vi "Create New Rubix Cube.vi"(8 "error out":errorcluster, 11 "Rubix Array pattern":string[][](array[string])) -> (0 "error out(no error)":errorcluster)   [LabVIEW 2019]
uses:
  Scene Commands.ctl
  Cube Data Ops.ctl
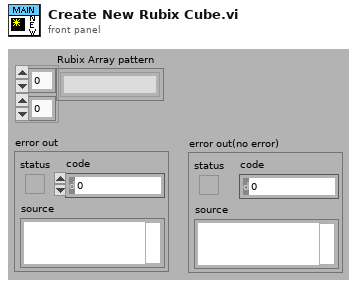
[diagram p1: front panel]
types:
  T1 = typedef "Scene Commands.ctl" = enum16{"Init", "Set Rubix Text Array", "Get Rubix Ref Array", "Generate Rubix Array", "Get Rubix Array", "Show Render Window", "Go To Face", "Rotate", "Update Scene", "Clear Rubix"}
  T2 = typedef "Cube Data Ops.ctl" = enum16{"Initialize", "Set Rubix Ref Array", "Set Rubix Text Array", "Set Current Face", "Get Rubix Text Array", "Generate Rubix Array", "Get Rubix array", "Get Facets to move", "Randomize", "Top row left", "Top row right", "Middle row left", "Middle row right", "Bottom row left", "Bottom row right", "Left column up", "Left column down", "Middle column up", "Middle column down", "Right column up", "Right column down", "Face ccw", "Face cw"}
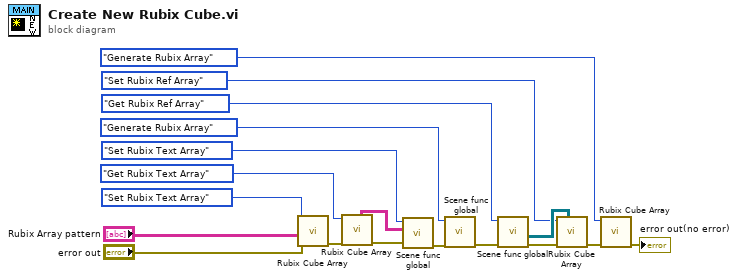
[diagram p0: block diagram]
diagram:
  n1 = call "Rubix Cube Array.vi"("error in (no error)"="error out", "Rubix Text Array in"="Rubix Array pattern", "Command"=Cube_Data_Ops."Set Rubix Text Array") -> ("error out(no error)"=w5:errorcluster)  [unwired: 4 in, 4 out]
  n2 = call "Rubix Cube Array.vi"("error in (no error)"=w5, "Command"=Cube_Data_Ops."Get Rubix Text Array") -> ("error out(no error)"=w6:errorcluster, "Rubix Text Array Out"=w8:string[][])  [unwired: 5 in, 3 out]
  n3 = call "Scene func global.vi"("error in (no error)"=w6, "Rubix Text Array"=w8, "Commands"=Scene_Commands."Set Rubix Text Array") -> ("error out"=w12:errorcluster)  [unwired: 7 in, 1 out]
  n4 = call "Scene func global.vi"("error in (no error)"=w12, "Commands"=Scene_Commands."Generate Rubix Array") -> ("error out"=w14:errorcluster)  [unwired: 8 in, 1 out]
  n5 = call "Scene func global.vi"("error in (no error)"=w14, "Commands"=Scene_Commands."Get Rubix Ref Array") -> ("error out"=w15:errorcluster, "Rubix ref Array"=w17:refnum<vi>[][])  [unwired: 8 in]
  n6 = call "Rubix Cube Array.vi"("Rubix ref Array"=w17, "error in (no error)"=w15, "Command"=Cube_Data_Ops."Set Rubix Ref Array") -> ("error out(no error)"=w10:errorcluster)  [unwired: 4 in, 4 out]
  n7 = call "Rubix Cube Array.vi"("error in (no error)"=w10, "Command"=Cube_Data_Ops."Generate Rubix Array") -> ("error out(no error)"=→"error out(no error)":errorcluster)  [unwired: 5 in, 4 out]
